vi "Keithley2200series_Start.vi"(0 "VISA resource name 2":refnum<visa-resource-name>, 1 "Function(0:Voltage) 3":u16(ring) items=["Voltage", "Current"], 2 "Out set 2":dbl, 3 "error in (no error)":errorcluster, 4 "Cml set 2":dbl) -> (5 "VISA out":refnum<visa-resource-name>, 6 "Meas Func":i32, 7 "error out 2":errorcluster)   [LabVIEW 2014]
uses:
  C:/Users/rad/Desktop/Keithley 2200 Series Power Supplies Ver 1.2 (LV2009)/Keithley 2200 Series/Keithley 2200 Series.lvlib
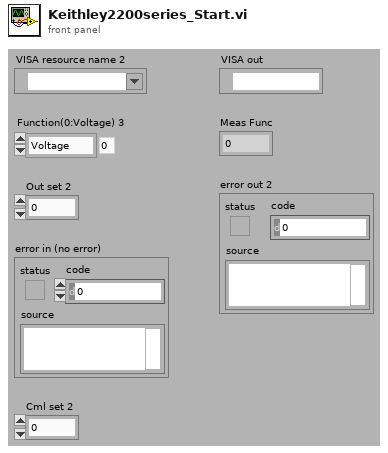
[diagram p1: front panel]
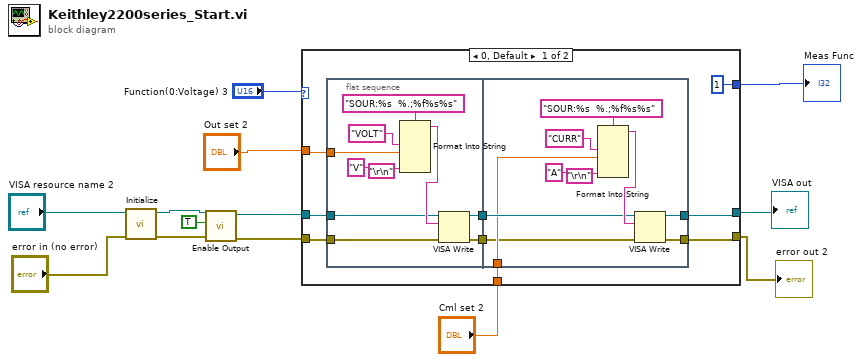
[diagram p0: block diagram]
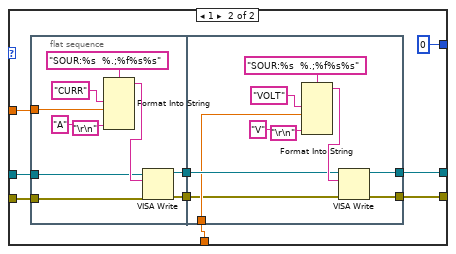
[diagram p2: hidden frame]
diagram:
  n1 = call "Initialize.vi"("error in (no error)"="error in (no error)", "VISA resource name"="VISA resource name 2") -> ("error out"=w3:errorcluster, "VISA resource name out"=w4:refnum<visa-resource-name>)  [unwired: 8 in]
  n2 = call "Enable Output.vi"("error in (no error)"=w3, "Enable Output (T: Enable)"=TRUE, "VISA resource name"=w4) -> ("error out"=w7:errorcluster, "VISA resource name out"=w8:refnum<visa-resource-name>)  [unwired: 7 out]
  n3 = case shown="0, Default" "Function(0:Voltage) 3" {
    tunnel: "Out set 2" -> [w22 w49]
    tunnel: "Cml set 2" -> [w20 w48]
    tunnel: w8 -> [w15 w47]
    tunnel: w7 -> [w14 w46]
    tunnel: [w18 w45] -> w6
    tunnel: [w17 w44] -> w5
    tunnel: [1 0] -> w13
    frame 0, Default {
      n4 = flat-sequence {
        tunnel: w22 -> [w30]
        tunnel: [w26] -> w21
        tunnel: [w25] -> w19
        tunnel: w15 -> [w24]
        tunnel: w14 -> [w23]
        tunnel: w21 -> [w37]
        tunnel: w20 -> [w36]
        tunnel: w19 -> [w35]
        tunnel: [w34] -> w18
        tunnel: [w33] -> w17
        frame #0 {
          n5 = Format Into String(format string="SOUR:%s  %.;%f%s%s", "VOLT" ("format string"), w30, "V" ("input 3"), "\r\n" ("End of Line Constant")) -> (resulting string=w27:string)  [unwired: 2 in, 1 out]
          n6 = VISA Write(VISA resource name=w24, write buffer=w27, error in (no error)=w23) -> (VISA resource name out=w26:refnum<visa-resource-name>, error out=w25:errorcluster)  [unwired: 1 out]
        }
        frame #1 {
          n7 = Format Into String(format string="SOUR:%s  %.;%f%s%s", "CURR" ("format string"), w36, "A" ("input 3"), "\r\n" ("End of Line Constant")) -> (resulting string=w38:string)  [unwired: 2 in, 1 out]
          n8 = VISA Write(VISA resource name=w37, write buffer=w38, error in (no error)=w35) -> (VISA resource name out=w34:refnum<visa-resource-name>, error out=w33:errorcluster)  [unwired: 1 out]
        }
      }
    }
    frame 1 {
      n9 = flat-sequence {
        tunnel: w49 -> [w59]
        tunnel: [w55] -> w51
        tunnel: [w54] -> w50
        tunnel: w47 -> [w53]
        tunnel: w46 -> [w52]
        tunnel: w51 -> [w66]
        tunnel: w48 -> [w65]
        tunnel: w50 -> [w64]
        tunnel: [w63] -> w45
        tunnel: [w62] -> w44
        frame #0 {
          n10 = Format Into String(format string="SOUR:%s  %.;%f%s%s", "CURR" ("format string"), w59, "A" ("input 3"), "\r\n" ("End of Line Constant")) -> (resulting string=w56:string)  [unwired: 2 in, 1 out]
          n11 = VISA Write(VISA resource name=w53, write buffer=w56, error in (no error)=w52) -> (VISA resource name out=w55:refnum<visa-resource-name>, error out=w54:errorcluster)  [unwired: 1 out]
        }
        frame #1 {
          n12 = Format Into String(format string="SOUR:%s  %.;%f%s%s", "VOLT" ("format string"), w65, "V" ("input 3"), "\r\n" ("End of Line Constant")) -> (resulting string=w67:string)  [unwired: 2 in, 1 out]
          n13 = VISA Write(VISA resource name=w66, write buffer=w67, error in (no error)=w64) -> (VISA resource name out=w63:refnum<visa-resource-name>, error out=w62:errorcluster)  [unwired: 1 out]
        }
      }
    }
  }
  "VISA out" <- w6
  "error out 2" <- w5
  "Meas Func" <- w13
